vi "Write Encoding.vi"(10 "Encoding":refnum<class "Encoding.lvclass">, 11 "ConfigManager in":refnum<class "ConfigManager.lvclass">) -> (3 "ConfigManager out":refnum<class "ConfigManager.lvclass">)   [LabVIEW 2013, in "CfgManager.lvlib" / "ConfigManager.lvclass"]
uses:
  ConfigManager.lvclass
  Encoding/Encoding.lvclass
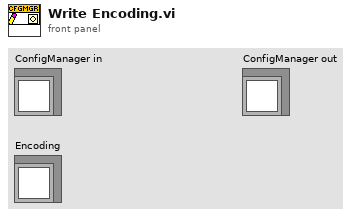
[diagram p1: front panel]
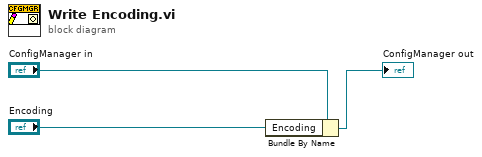
[diagram p0: block diagram]
diagram:
  n1 = Bundle By Name(cluster="ConfigManager in", "Encoding"="Encoding") -> (→"ConfigManager out":refnum<class "ConfigManager.lvclass">)
